vi "Test Generate Mock Class Replaces Class Control and Constant.vi"(8 "error in (no error)":errorcluster, 11 "Test Case In":refnum<class "Pure Mock Class Generator Test.lvclass">) -> (0 "error out":errorcluster, 3 "Test Case Out":refnum<class "Pure Mock Class Generator Test.lvclass">)   [LabVIEW 2020, in "Pure Mock Class Generator Test.lvclass"]
uses:
  Pure Mock Class Generator Test.lvclass
  <vilib>/Astemes/LUnit/Test Case.lvclass
  source/Scripting/Pure Mock Class Generator/Pure Mock Class Generator.lvclass
  C:/Program Files (x86)/National Instruments/LabVIEW 2020/vi.lib/Astemes/LUnit/Test Case.lvclass
panel:
  out "No error?":bool
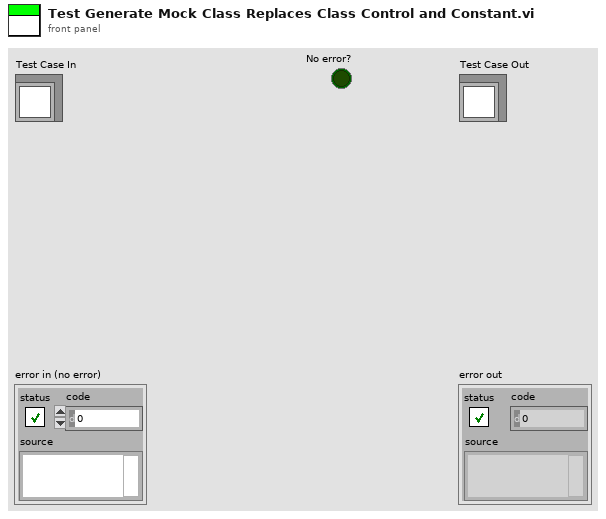
[diagram p1: front panel]
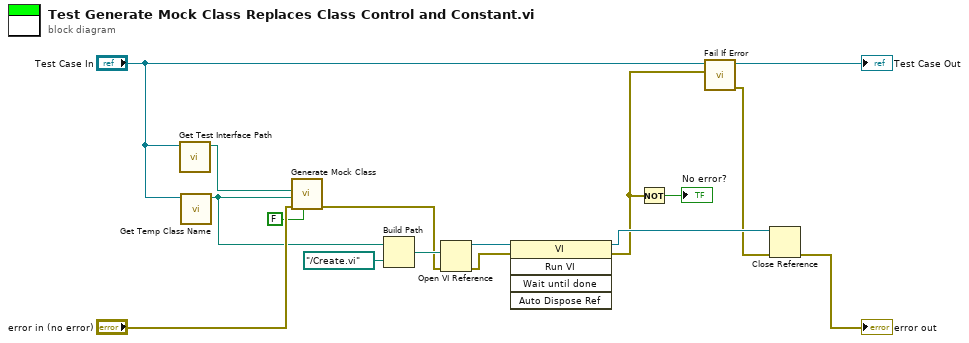
[diagram p0: block diagram]
diagram:
  n1 = call "Get Test Interface Path.vi"("Mock Class Generator Test in"="Test Case In") -> ("Test Class Path"=w15:path)  [unwired: 10 in]
  n2 = call "Get Temp Class Name.vi"("Mock Class Generator Test in"="Test Case In") -> ("Test Class Path"=w11:path)  [unwired: 10 in]
  n3 = call "Generate Mock Class.vi"("Add to lvproj?"=FALSE, "error in (no error)"="error in (no error)", "Destination Class Path"=w11, "Source Class Path"=w15) -> ("error out"=w6:errorcluster)  [unwired: 7 in]
  n4 = Build Path(base path=w11, name or relative path=path "../Create.vi") -> (appended path=w9:path)
  n5 = Open VI Reference(vi path=w9, error in (no error)=w6) -> (vi reference=w8:refnum<vi>, error out=w7:errorcluster)  [unwired: 4 in]
  n6 = invoke class="VI" method="Run VI"(reference=w8, error in=w7) -> (reference out=w5:refnum<vi>, error out=w2:errorcluster)  [unwired: 3 in, 3 out]
  n7 = Not(x=w2) -> (.not. x?=→"No error?":bool)
  n8 = call <vilib>:"Fail If Error.vi"("Assert error"=w2, "LUnit Test Case In"="Test Case In") -> ("error out"=w4:errorcluster, "LUnit Test Case Out"=→"Test Case Out":refnum<class "Pure Mock Class Generator Test.lvclass">)  [unwired: 8 in]
  n9 = Close Reference(reference=w5, error in (no error)=w4) -> (error out=→"error out":errorcluster)
